vi "Navigating Nodes and Wires.vi"   [LabVIEW 2023]
doc: "This VI searches for One Button Dialog functions in a target VI. If it finds a One Button Dialog function, it changes the text of the button to say \"Okay!\"\n\nThe Detailed Help explains how this example illustrates a general procedure for using a reference to a node to obtain a reference to a connected wire. Furthermore, the Detailed Help links to other navigation techniques that this example illustrates, including navigating from a wire to a node."
uses:
  <vilib>/Utility/traverseref.llb/TRef TravTarget.ctl
  <vilib>/Utility/traverseref.llb/VI Scripting - Traverse.lvlib
panel:
  # "Select Help>>Show Context Help and move the cursor over the VI icon to display help for this VI.\n\nBefore you start: Open the Detailed Help for this example to display the Navigating from a Node to a Wire Using VI Scripting topic in the  LabVIEW Help. That topic provides additional details about how this example illustrates the general procedure for using a reference to a node to obtain a reference to a connected wire. That topic also provides links to other navigation techniques that this example illustrates, including navigating from a wire to a node.\n\nThis VI searches for One Button Dialog functions in a target VI. If it finds a One Button Dialog function, it changes the text of the button to say \"Okay!\".\n\nOpen the target VI to observe the effects of this scripting VI. The default target VI is located in labview\\examples\\Application Control\\VI Scripting\\Finding and Modifying Objects.\n\nTo run this VI more than once, close the target VI and do not save changes."
  # "Overview: Demonstrates the use of VI Scripting to programmatically detect and modify the value of a specific block diagram constant.\nInstructions:\n1. Open Test - Navigating Nodes and Wires Target.vi.\n2. Run this VI. Observe the change to the value of the block diagram constant within the Test VI."
types:
  T1 = typedef "TRef TravTarget.ctl" = enum16{"FP", "BD", "Other"}
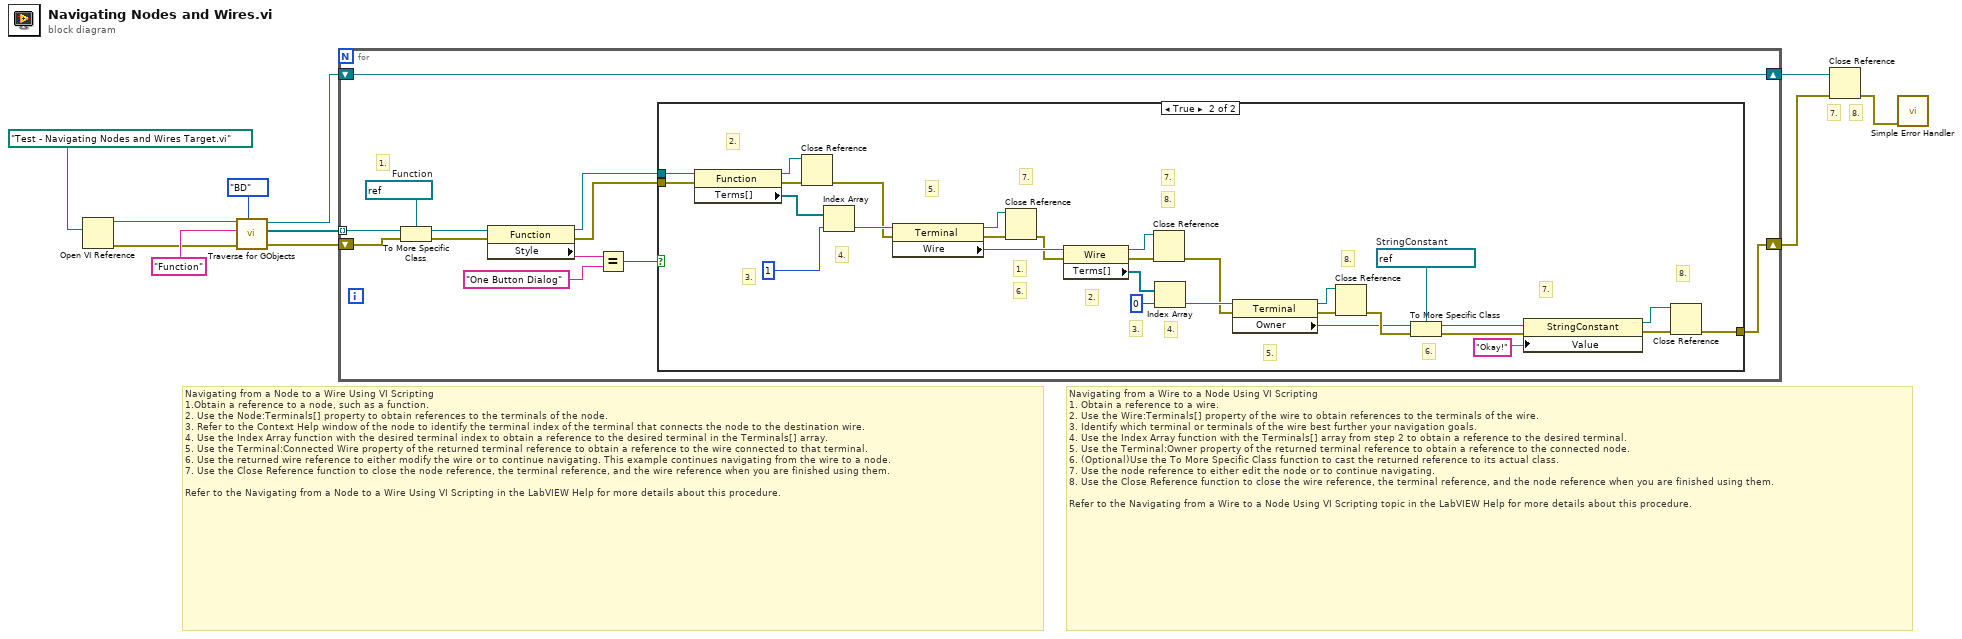
[diagram p0: block diagram]
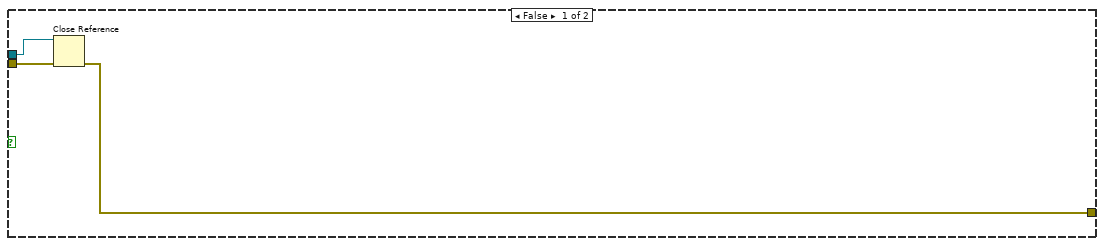
[diagram p2: hidden frame]
diagram:
  # "8."
  # "7."
  # "Navigating from a Wire to a Node Using VI Scripting\n1. Obtain a reference to a wire.\n2. Use the Wire:Terminals[] property of the wire to obtain references to the terminals of the wire.\n3. Identify which terminal or terminals of the wire best further your navigation goals.\n4. Use the Index Array function with the Terminals[] array from step 2 to obtain a reference to the desired terminal.\n5. Use the Terminal:Owner property of the returned terminal reference to obtain a reference to the connected node.\n6. (Optional)Use the To More Specific Class function to cast the returned reference to its actual class.\n7. Use the node reference to either edit the node or to continue navigating.\n8. Use the Close Reference function to close the wire reference, the terminal reference, and the node reference when you are finished using them.\n\nRefer to the Navigating from a Wire to a Node Using VI Scripting topic in the LabVIEW Help for more details about this procedure."
  # "Navigating from a Node to a Wire Using VI Scripting\n1.Obtain a reference to a node, such as a function.\n2. Use the Node:Terminals[] property to obtain references to the terminals of the node.\n3. Refer to the Context Help window of the node to identify the terminal index of the terminal that connects the node to the destination wire.\n4. Use the Index Array function with the desired terminal index to obtain a reference to the desired terminal in the Terminals[] array.\n5. Use the Terminal:Connected Wire property of the returned terminal reference to obtain a reference to the wire connected to that terminal.\n6. Use the returned wire reference to either modify the wire or to continue navigating. This example continues navigating from the wire to a node.\n7. Use the Close Reference function to close the node reference, the terminal reference, and the wire reference when you are finished using them.\n\nRefer to the Navigating from a Node to a Wire Using VI Scripting in the LabVIEW Help for more details about this procedure."
  n1 = Open VI Reference(vi path=path "Test - Navigating Nodes and Wires Target.vi") -> (vi reference=w7:refnum<vi>, error out=w2:errorcluster)  [unwired: 5 in]
  n2 = call <vilib>:"Traverse for GObjects.vi"("Traverse Target"=TRef_TravTarget."BD", "error in (no error)"=w2, "Class Name"="Function", "VI Refnum"=w7) -> ("error out"=w8:errorcluster, "References"=w6:refnum<vi>[], "dup VI Refnum"=w3:refnum<vi>)  [unwired: 4 in, 1 out]
  n3 = for {
    tunnel: w6 -> [w23] mode=indexing
    shift-right: [w13] -> w4
    shift-left: w8 -> [w14]
    shift-right: [w12] -> w5
    shift-left: w3 -> [w12]
    w22 = refnum<vi> refnum  # Function
    # "1."
    n4 = To More Specific Class(target class=w22, reference=w23, error in=w14) -> (specific class reference=w21:refnum<vi>, error out=w20:errorcluster)
    n5 = property on="Property Node" class="Function"(reference=w21, error in=w20) -> (reference out=w16:refnum<vi>, error out=w15:errorcluster, "Style"=w19:string)
    n6 = Equal?(x=w19, y="One Button Dialog") -> (x = y?=w17:bool)
    n7 = case shown="True" w17 {
      tunnel: w16 -> [w25 w36]
      tunnel: w15 -> [w26 w35]
      tunnel: [w24 w27] -> w13
      frame False {
        n8 = Close Reference(reference=w25, error in (no error)=w26) -> (error out=w24:errorcluster)
      }
      frame True {
        w45 = refnum<vi> refnum  # StringConstant
        # "3."
        # "8."
        # "8."
        # "8."
        # "7."
        # "6."
        # "5."
        # "4."
        # "3."
        # "2."
        # "1."
        # "7."
        # "7."
        # "6."
        # "5."
        # "4."
        # "2."
        n9 = property on="Property Node" class="Function"(reference=w36, error in=w35) -> (reference out=w34:refnum<vi>, error out=w33:errorcluster, "Terms[]"=w37:refnum<vi>[])
        n10 = Close Reference(reference=w34, error in (no error)=w33) -> (error out=w32:errorcluster)
        n11 = Index Array(array=w37, index=1) -> (element=w39:refnum<vi>)
        n12 = property on="Property Node" class="Terminal"(reference=w39, error in=w32) -> (reference out=w43:refnum<vi>, error out=w51:errorcluster, "Wire"=w40:refnum<vi>)
        n13 = Close Reference(reference=w43, error in (no error)=w51) -> (error out=w29:errorcluster)
        n14 = property on="Property Node" class="Wire"(reference=w40, error in=w29) -> (reference out=w31:refnum<vi>, error out=w30:errorcluster, "Terms[]"=w41:refnum<vi>[])
        n15 = Close Reference(reference=w31, error in (no error)=w30) -> (error out=w28:errorcluster)
        n16 = Index Array(array=w41, index=0) -> (element=w49:refnum<vi>)
        n17 = property on="Property Node" class="Terminal"(reference=w49, error in=w28) -> (reference out=w54:refnum<vi>, error out=w53:errorcluster, "Owner"=w44:refnum<vi>)
        n18 = Close Reference(reference=w54, error in (no error)=w53) -> (error out=w55:errorcluster)
        n19 = To More Specific Class(target class=w45, reference=w44, error in=w55) -> (specific class reference=w46:refnum<vi>, error out=w47:errorcluster)
        n20 = property on="Property Node" class="StringConstant"(reference=w46, error in=w47, "Value"="Okay!") -> (reference out=w52:refnum<vi>, error out=w50:errorcluster)
        n21 = Close Reference(reference=w52, error in (no error)=w50) -> (error out=w27:errorcluster)
      }
    }
  }
  n22 = Close Reference(reference=w5, error in (no error)=w4) -> (error out=w1:errorcluster)
  n23 = call <vilib>:"Simple Error Handler.vi"("error in (no error)"=w1) -> ()  [unwired: 4 in, 5 out]
